vi "Periodic Tasks.vi"(8 "error in":errorcluster) -> ()   [LabVIEW 2014]
doc: "This VI runs in parallel to other tasks. It can contain as many user-defined periodic loops as you need. These can carry out PID or other sorts of timed response."
uses:
  <vilib>/Rock Robotics/WPI/Joystick/WPI_JoystickGetSetRefNum.vi
  <vilib>/Rock Robotics/WPI/RobotDrive/WPI_RobotDriveGetSetRefNum.vi
  <vilib>/Rock Robotics/Network Tables/SD Write Numeric Array.vi
panel:
  out "Result 6":dbl
  out "Result 5":dbl
  out "Sine 2":dynamicdata(graph) caption="Sine"
  out "Sine":dynamicdata(graph)
  out "Result 4":dynamicdata(graph) caption="Result"
  out "Result 3":dynamicdata(graph) caption="Result"
  in  "Angle":dbl
  out "Result 2":dynamicdata(graph) caption="Result"
  out "Result":dynamicdata(graph)
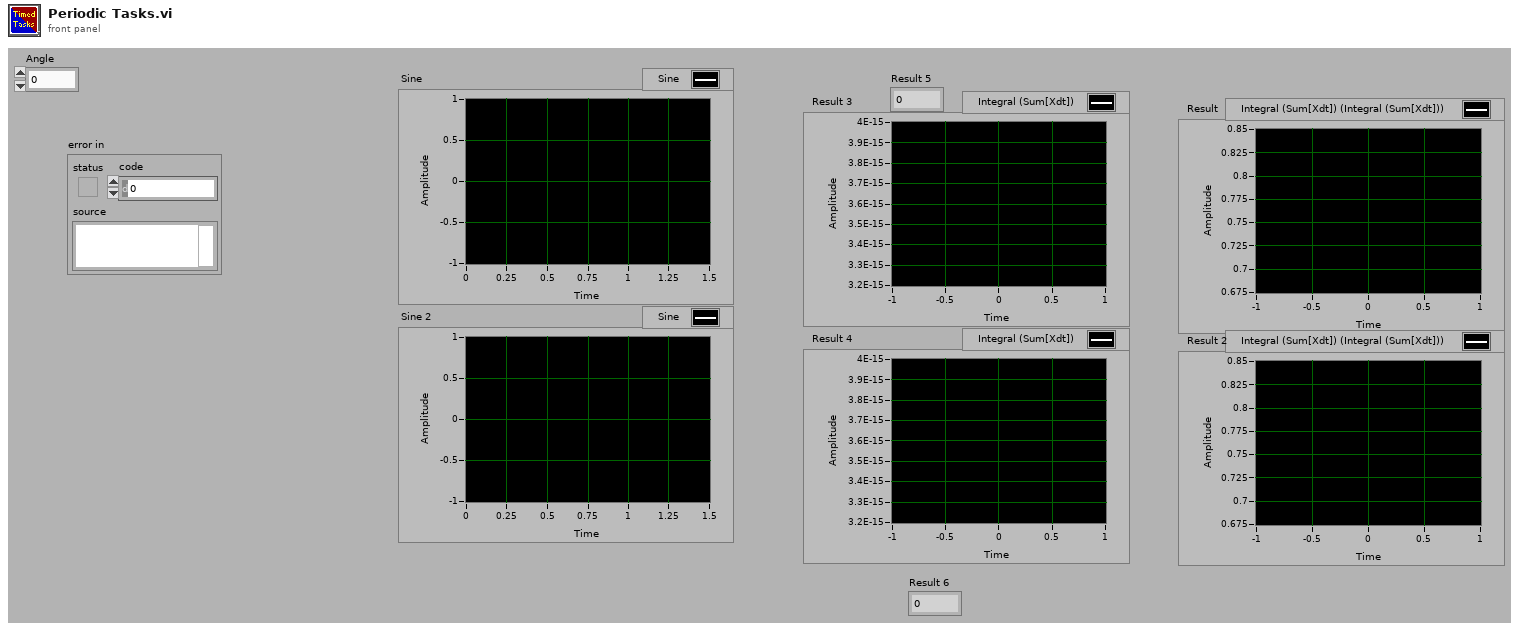
[diagram p1: front panel]
types:
  T1 = typedef "WPI_JoystickDevRef.ctl" = cluster{"Device":T2}
  T2 = typedef "WPI_JoystickDeviceEnum.ctl" = enum16{"USB 0", "USB 1", "USB 2", "USB 3", "USB 4", "USB 5"}
  T3 = typedef "WPI_RobotDriveDevRef.ctl" = cluster{"DevStatus":errorcluster, "Motors[]":T4[], "Square Inputs":bool, "Max Output":dbl}
  T4 = typedef "WPI_MotorControlDeviceRef.ctl" = cluster{"DeviceStatus":errorcluster, "Type":T5, "PWM":cluster{"Controller":T6, "PWM Channel":T7, "DeadBand":T8}, "CAN":cluster{"Device Number":u8, "Control Mode":T9, "Semaphore":T10, "Max Vout":dbl, "TalonSRX Control Mode":T11}, "Invert":bool, "TransformRef":T12, "InvTransformRef":T12}
  T5 = typedef "WPI_MotorControlType.ctl" = enum16{"PWM", "CAN", "CANTalonSRX"}
  T6 = typedef "FPGA_TypedefDigitalModule.ctl" = enum16{"Controller 1"}
  T7 = typedef "FPGA_DIOPWMChannel.ctl" = enum8{"PWM 0", "PWM 1", "PWM 2", "PWM 3", "PWM 4", "PWM 5", "PWM 6", "PWM 7", "PWM 8", "PWM 9", "PWM MXP 0", "PWM MXP 1", "PWM MXP 2", "PWM MXP 3", "PWM MXP 4", "PWM MXP 5", "PWM MXP 6", "PWM MXP 7", "PWM MXP 8", "PWM MXP 9", "Invalid"}
  T8 = typedef "WPI_PWMDeadband.ctl" = cluster{"Name":string, "maxPositivePwm":i32, "minPositivePwm":i32, "centerPwm":i32, "maxNegativePwm":i32, "minNegativePwm":i32, "angularRange":u16}
  T9 = typedef "WPI_CANJaguar_ControlMode.ctl" = enum8{"Percent VBus", "Current", "Speed", "Position", "Voltage"}
  T10 = typedef "Semaphore RefNum" = refnum<k1>
  T11 = typedef "WPI_CANTalonSRX_APIControlMode.ctl" = enum8{"Percent VBus", "Speed", "Position", "Slave", "Unchanged / Invalid"}
  T12 = typedef "WPI_PWMTransform_ConPane.ctl" = refnum<vi>
  T13 = cluster{"JoystickDevRef":T1, "RobotDriveDevRef":T3}
  T14 = cluster{"roboRIO input current (A)":dbl, "voltage (V)":dbl, "current (A)":dbl, "current (A)":dbl, "current (A)":dbl, "current (A)":dbl, "current (A)":dbl, "current (A)":dbl, "current (A)":dbl}
  T15 = typedef "WPI_AccelerometerDevRef.ctl" = cluster{"DevStatus":errorcluster, "Controller":T16, "Scaling":T17, "Analog Channels":T18, "I2C Bus":T20, "SPI Bus":T21, "Accel Range":T22, "ADXL345 Axes":T23, "Handle":i32, "Device Address":u8, "Accel Type":enum16{"Analog", "ADXL345 I2C", "ADXL345 SPI", "Internal"}}
  T16 = typedef "FPGA_TypedefAnalogModule.ctl" = enum16{"Controller 1"}
  T17 = typedef "WPI_AccelerometerScaling.ctl" = cluster{"Gain (VoltsPerG)":dbl, "Center Voltage":dbl}
  T18 = typedef "WPI_AccelerometerAnalogChannels.ctl" = cluster{"X-Axis":T19, "Y-Axis":T19, "Z-Axis":T19}
  T19 = typedef "FPGA_AIChannel.ctl" = enum8{"AI 0", "AI 1", "AI 2", "AI 3", "AI MXP 0", "AI MXP 1", "AI MXP 2", "AI MXP 3", "Invalid"}
  T20 = typedef "i2c_bus.ctl" = enum16{"I2C On-Board", "I2C MXP", "Invalid"}
  T21 = typedef "spi_bus.ctl" = enum16{"SPI On-Board, CS0", "SPI On-Board, CS1", "SPI On-Board, CS2", "SPI On-Board, CS3", "SPI MXP", "Invalid"}
  T22 = typedef "ADXL345 Range.ctl" = u8
  T23 = typedef "WPI_AccelerometerADXL345 Axes.ctl" = cluster{"X-Axis":bool, "Y-Axis":bool, "Z-Axis":bool}
  T24 = typedef "WPI_GyroDevRef.ctl" = cluster{"DevStatus":errorcluster, "Analog Module":T16, "Analog Channel":T19, "Offset":dbl, "Gain (VoltsPerDegree/Second)":dbl}
  T25 = cluster{"X-Axis":dbl, "Y-Axis":dbl, "Z-Axis":dbl}
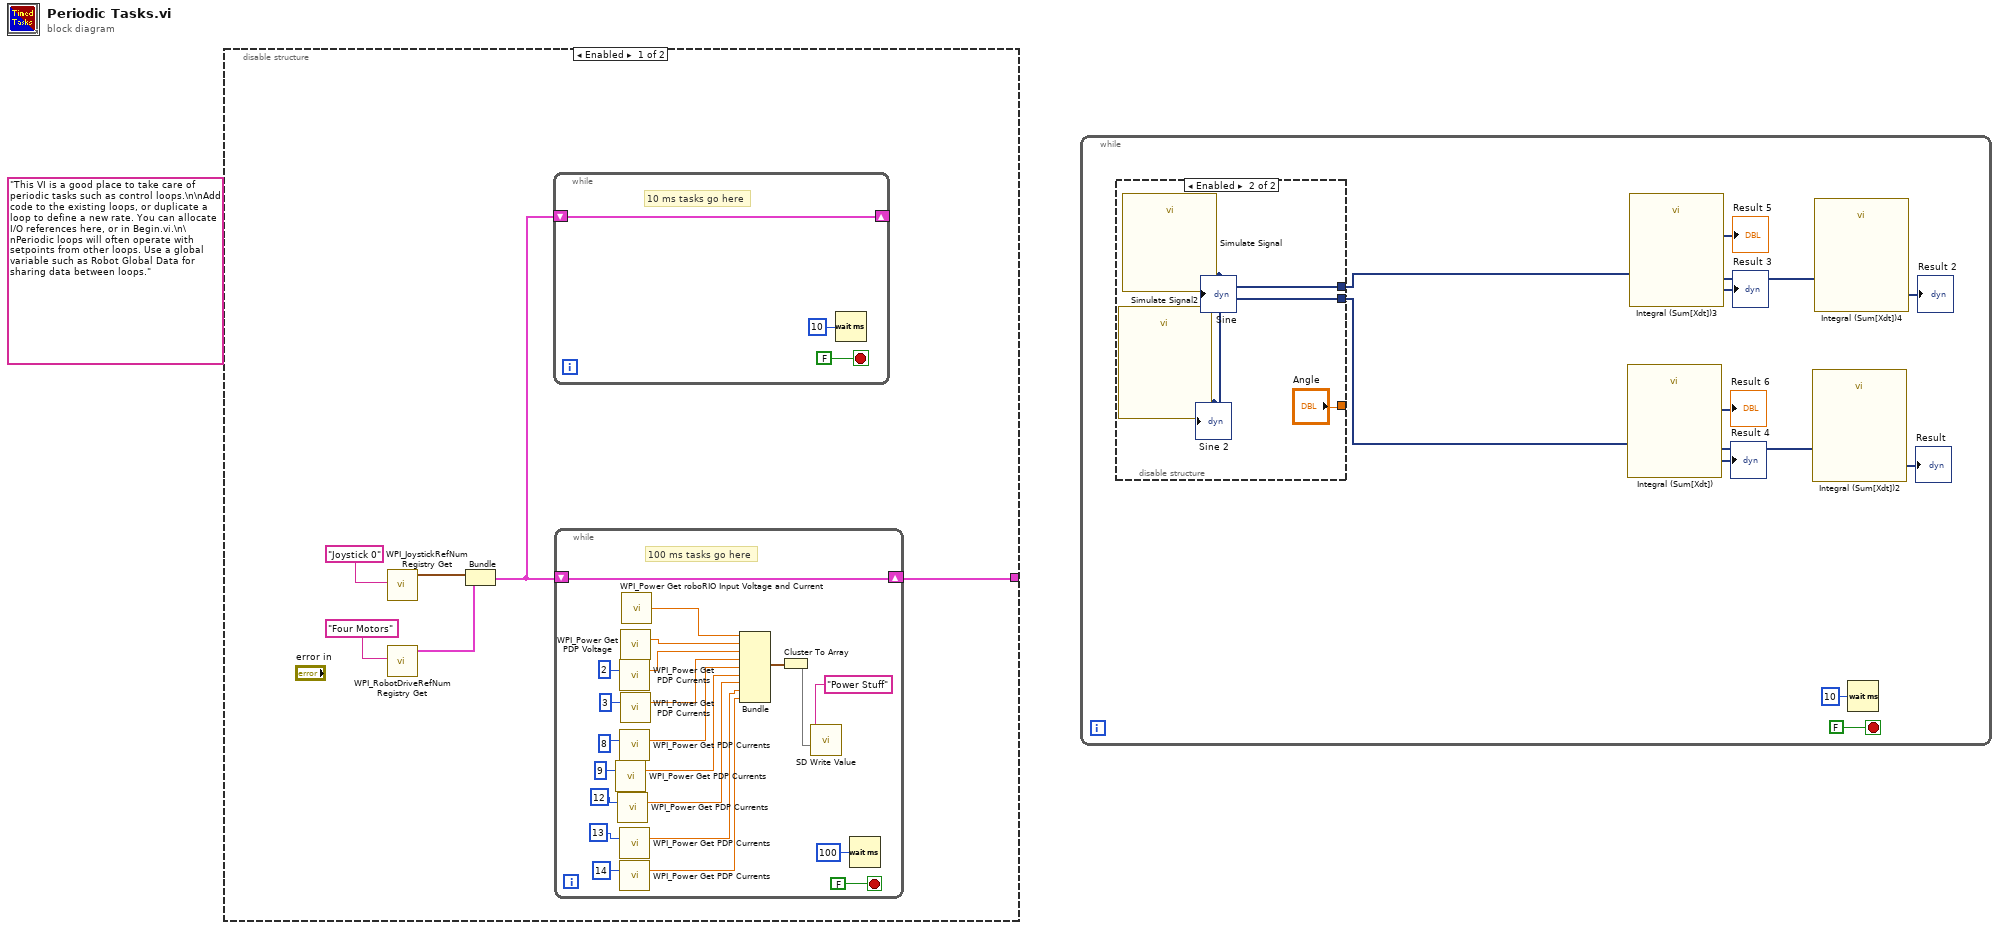
[diagram p0: block diagram]
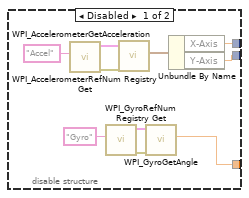
[diagram p3: hidden frame]
diagram:
  (unwired) "This VI is a good place to take care of periodic tasks such as control loops.\n\nAdd code to the existing loops, or duplicate a loop to define a new rate. You can allocate I/O references here, or in Begin.vi.\n\nPeriodic loops will often operate with setpoints from other loops. Use a global variable such as Robot Global Data for sharing data between loops."
  n1 = disable-structure shown="Enabled" {
    disable-tunnel: [w1 _] -> _
    frame Enabled {
      n2 = call <vilib>:"WPI_JoystickRefNum Registry Get.vi"("refnum name"="Joystick 0") -> ("JoystickDevRef"=w4:T1)  [unwired: 1 in, 9 out]
      n3 = call <vilib>:"WPI_RobotDriveRefNum Registry Get.vi"("refnum name"="Four Motors") -> ("RobotDriveDevRef"=w3:T3)  [unwired: 1 in, 9 out]
      n4 = Bundle("JoystickDevRef"=w4, "RobotDriveDevRef"=w3) -> (w2:T13)  [unwired: 1 out]
      n5 = while {
        shift-right: [w29] -> _
        shift-left: w2 -> [w29]
        stop <- FALSE stop-if-true
        # "10 ms tasks go here"
        n6 = Wait (ms)(milliseconds to wait=u32 10) -> ()  [unwired: 1 out]
      }
      n7 = while {
        shift-right: [w26] -> w1
        shift-left: w2 -> [w26]
        stop <- FALSE stop-if-true
        # "100 ms tasks go here"
        n8 = call <vilib>:"WPI_Power Get PDP Currents.vi"("PDP Channel"=9) -> ("current (A)"=w14:dbl)  [unwired: 12 in, 2 out]
        n9 = call <vilib>:"WPI_Power Get PDP Currents.vi"("PDP Channel"=12) -> ("current (A)"=w13:dbl)  [unwired: 12 in, 2 out]
        n10 = call <vilib>:"WPI_Power Get PDP Currents.vi"("PDP Channel"=2) -> ("current (A)"=w17:dbl)  [unwired: 12 in, 2 out]
        n11 = call <vilib>:"WPI_Power Get PDP Currents.vi"("PDP Channel"=8) -> ("current (A)"=w15:dbl)  [unwired: 12 in, 2 out]
        n12 = call <vilib>:"WPI_Power Get PDP Currents.vi"("PDP Channel"=13) -> ("current (A)"=w12:dbl)  [unwired: 12 in, 2 out]
        n13 = call <vilib>:"WPI_Power Get PDP Currents.vi"("PDP Channel"=14) -> ("current (A)"=w11:dbl)  [unwired: 12 in, 2 out]
        n14 = call <vilib>:"WPI_Power Get PDP Voltage.vi"() -> ("voltage (V)"=w18:dbl)  [unwired: 14 in, 1 out]
        n15 = call <vilib>:"WPI_Power Get PDP Currents.vi"("PDP Channel"=3) -> ("current (A)"=w16:dbl)  [unwired: 12 in, 2 out]
        n16 = call <vilib>:"WPI_Power Get roboRIO Input Voltage and Current.vi"() -> ("roboRIO input current (A)"=w10:dbl)  [unwired: 13 in, 2 out]
        n17 = Bundle("roboRIO input current (A)"=w10, "voltage (V)"=w18, "current (A)"=w17, "current (A)"=w16, "current (A)"=w15, "current (A)"=w14, "current (A)"=w13, "current (A)"=w12, "current (A)"=w11) -> (w9:T14)  [unwired: 1 in]
        n18 = Cluster To Array(cluster=w9) -> (array=w8:dbl[])
        n19 = call-poly <vilib>:"SD Write Value.vi"("Numeric Array"=w8, "Name"="Power Stuff") -> ()  [unwired: 8 in, 2 out]
        n20 = Wait (ms)(milliseconds to wait=u32 100) -> ()  [unwired: 1 out]
      }
    }
    frame Disabled {
    }
  }
  n21 = while {
    stop <- FALSE stop-if-true
    n22 = disable-structure shown="Enabled" {
      disable-tunnel: [w42 w51] -> w33
      disable-tunnel: [w41 w52] -> w32
      disable-tunnel: [w40 "Angle"] -> _
      frame Disabled {
        n23 = call <vilib>:"WPI_AccelerometerRefNum Registry Get.vi"("refnum name"="Accel") -> ("error out"=w48:errorcluster, "AccelerometerDevRef"=w49:T15)  [unwired: 9 in]
        n24 = call <vilib>:"WPI_GyroRefNum Registry Get.vi"("refnum name"="Gyro") -> ("error out"=w44:errorcluster, "GyroDevRef"=w43:T24)  [unwired: 9 in]
        n25 = call <vilib>:"WPI_AccelerometerGetAcceleration.vi"("error in"=w48, "AccelerometerDevRef"=w49) -> ("Accelerations"=w47:T25)  [unwired: 7 in, 2 out]
        n26 = call <vilib>:"WPI_GyroGetAngle.vi"("error in (no error)"=w44, "GyroDevRef"=w43) -> ("Angle"=w40:dbl)  [unwired: 6 in, 3 out]
        n27 = Unbundle By Name(w47) -> ("X-Axis"=w42:dbl, "Y-Axis"=w41:dbl)
      }
      frame Enabled {
        n28 = call "Simulate Signal2"() -> ("Sine"=w52:dynamicdata)  [unwired: 14 in, 1 out]
        "Sine 2" <- w52
        n29 = call "Simulate Signal"() -> ("Sine"=w51:dynamicdata)  [unwired: 14 in, 1 out]
        "Sine" <- w51
      }
    }
    n30 = call "Integral (Sum[Xdt])"("Signals"=w32) -> ("Result"=w37:dynamicdata)  [unwired: 5 in, 1 out]
    "Result 4" <- w37
    "Result 6" <- w37
    n31 = call "Integral (Sum[Xdt])3"("Signals"=w33) -> ("Result"=w36:dynamicdata)  [unwired: 5 in, 1 out]
    "Result 3" <- w36
    "Result 5" <- w36
    n32 = call "Integral (Sum[Xdt])2"("Signals"=w37) -> ("Result"=→"Result":dynamicdata)  [unwired: 5 in, 1 out]
    n33 = call "Integral (Sum[Xdt])4"("Signals"=w36) -> ("Result"=→"Result 2":dynamicdata)  [unwired: 5 in, 1 out]
    n34 = Wait (ms)(milliseconds to wait=u32 10) -> ()  [unwired: 1 out]
  }
